vi "Parallel Execution B.vi"() -> (0 "error out B":errorcluster)   [LabVIEW 2020]
panel:
  out "Iterations B":i32
  in  "Write Value B":dbl=1.5 format="%.6f"
  in  "Write Name B":string="DAC0"
  in  "stop":bool
  out "Error String B":string
  out "Read Value B":dbl format="%.6f"
  in  "Read Name B":string="AIN0"
  out "ConnectionType Out":i32
  out "DeviceType Out":i32
  in  "Identifier":string="470013239"
  in  "ConnectionType":string="usb"
  in  "DeviceType":string="t7"
  # "See comments on A example."
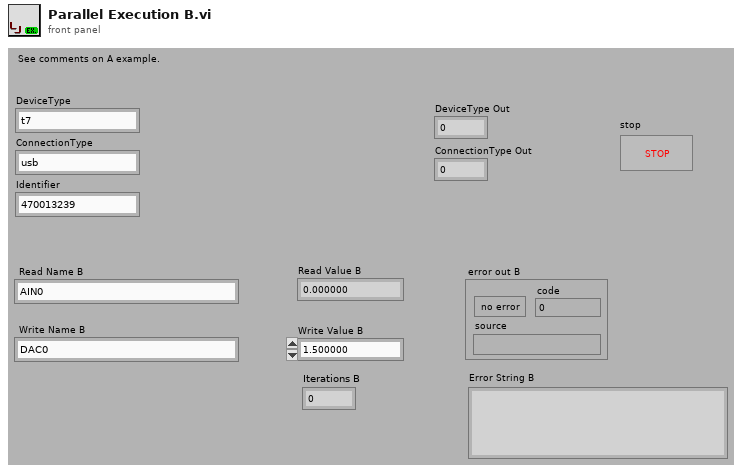
[diagram p1: front panel]
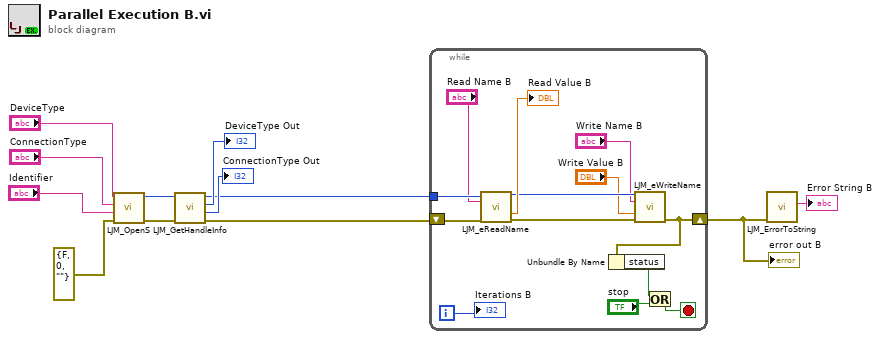
[diagram p0: block diagram]
diagram:
  n1 = call "LJM_OpenS.vi"("error in"=errorcluster {"status"=FALSE, "code"=0, "source"=""} ("error in (no error)"), "Identifier"="Identifier", "ConnectionType"="ConnectionType", "DeviceType"="DeviceType") -> ("error out"=w11:errorcluster, "Handle"=w10:i32)  [unwired: 6 in]
  n2 = call "LJM_GetHandleInfo.vi"("error in"=w11, "Handle In"=w10) -> ("error out"=w1:errorcluster, "ConnectionType"=→"ConnectionType Out":i32, "DeviceType"=→"DeviceType Out":i32, "Handle Out"=w2:i32)  [unwired: 2 in, 4 out]
  n3 = while {
    tunnel: w2 -> [w24]
    shift-right: [w17] -> w3
    shift-left: w1 -> [w25]
    i -> [w13]
    stop <- w21 stop-if-true
    n4 = call "LJM_eReadName.vi"("Handle In"=w24, "Name"="Read Name B", "error in"=w25) -> ("Handle Out"=w16:i32, "Value"=→"Read Value B":dbl, "error out"=w18:errorcluster)  [unwired: 10 in]
    n5 = call "LJM_eWriteName.vi"("Handle In"=w16, "Name"="Write Name B", "Value"="Write Value B", "error in"=w18) -> ("error out"=w17:errorcluster)  [unwired: 10 in, 1 out]
    n6 = Unbundle By Name(w17) -> ("status"=w19:bool)
    n7 = Or(x=w19, y="stop") -> (x .or. y?=w21:bool)
    "Iterations B" <- w13
  }
  "error out B" <- w3
  n8 = call "LJM_ErrorToString.vi"("error in"=w3) -> ("String"=→"Error String B":string)  [unwired: 10 in]
